vi "wav_reader.vi"() -> ()   [LabVIEW 2020]
panel:
  out "Waveform Chart":waveform(dbl)(graph)
  out "Waveform Graph":waveform(dbl)(graph)
  in  "path":path
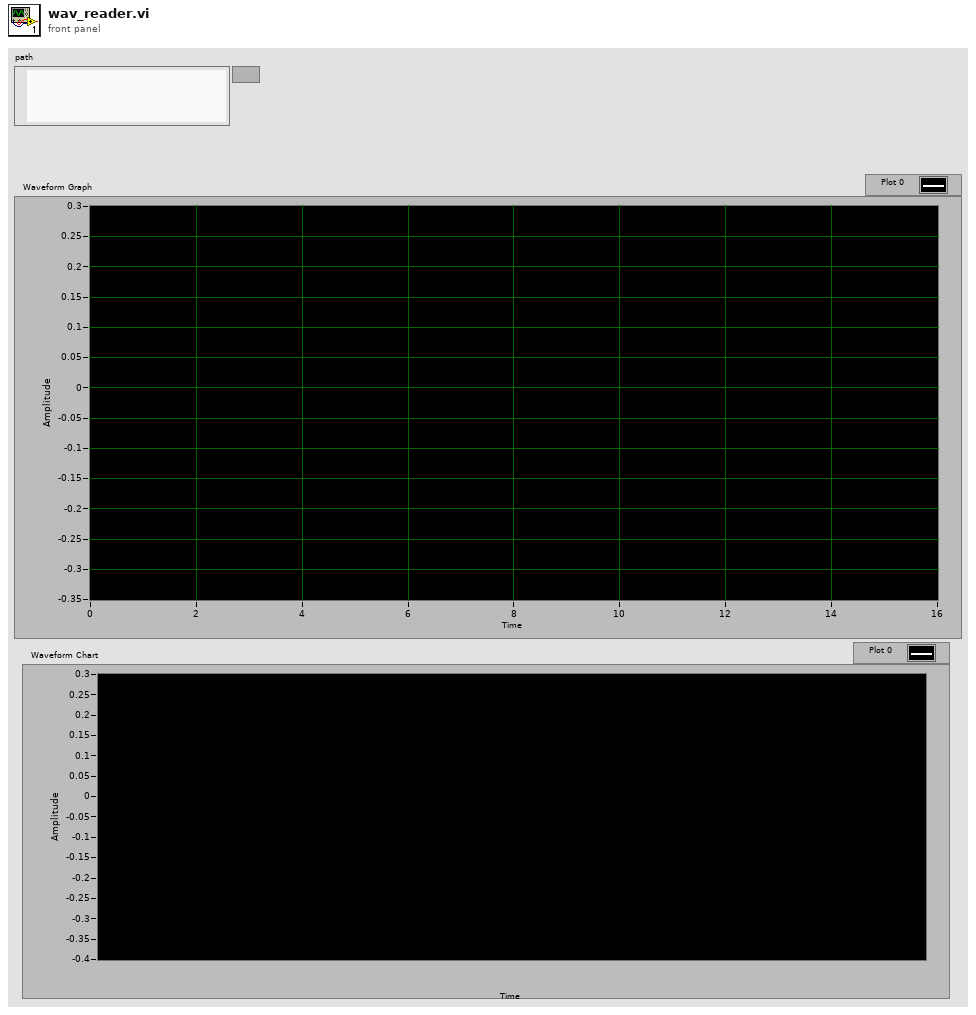
[diagram p1: front panel]
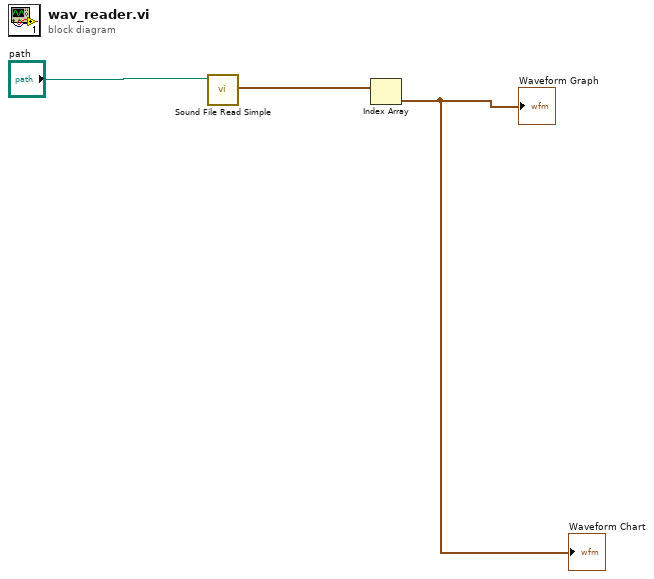
[diagram p0: block diagram]
diagram:
  n1 = call <vilib>:"Sound File Read Simple.vi"("path"="path") -> ("data"=w2:waveform(dbl)[])  [unwired: 7 in, 3 out]
  n2 = Index Array(array=w2) -> (element=→"Waveform Graph" →"Waveform Chart":waveform(dbl))  [unwired: 1 in]
